vi "New Hardware Selected.vi"(10 "error in (no error)":errorcluster, 11 "Hardware Index":i32) -> (2 "error out":errorcluster)   [LabVIEW 2020, in "RxnRover.lvlib"]
doc: "Fires the Update VI List Event with the provided Controller Array."
uses:
  RxnRover.lvlib
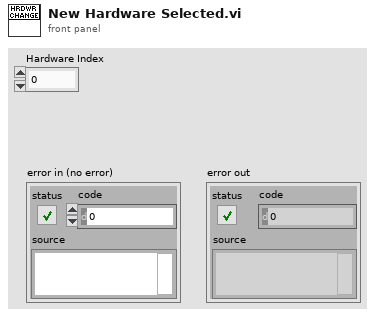
[diagram p1: front panel]
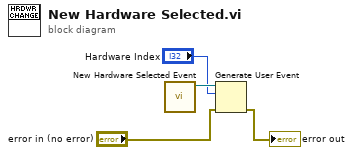
[diagram p0: block diagram]
diagram:
  n1 = call "New Hardware Selected Event.vi"() -> ("Hardware Index"=w4:refnum<user-event>)  [unwired: 11 in]
  n2 = Generate User Event(user event=w4, event data cluster="Hardware Index", error in="error in (no error)") -> (error out=→"error out":errorcluster)  [unwired: 1 in, 1 out]
